vi "subpanelGoToNode.vi"(8 "error in (no error)":errorcluster, 10 "Node Path":string, 11 "xceNode in":refnum<class "xceNode.lvclass">) -> (0 "error out":errorcluster, 2 "goToNode* out":refnum<data-value>, 3 "xceNode out":refnum<class "xceNode.lvclass">)   [LabVIEW 2013, in "xceNode.lvclass"]
doc: "Community access GoToNode method. This is nescessary to give permission to xceSubpanel to this method without making it public."
uses:
  xceNode.lvclass
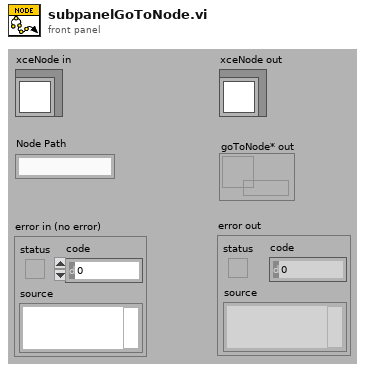
[diagram p1: front panel]
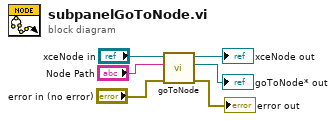
[diagram p0: block diagram]
diagram:
  n1 = call "goToNode.vi"("error in (no error)"="error in (no error)", "Node Path"="Node Path", "xceNode in"="xceNode in") -> ("error out"=→"error out":errorcluster, "goToNode* out"=→"goToNode* out":refnum<data-value>, "xceNode out"=→"xceNode out":refnum<class "xceNode.lvclass">)  [unwired: 6 in]
